vi "Poly_One_Text_Get.vi"(6 "Password?":bool, 7 "Text":string caption="Input Text", 8 "error in":errorcluster, 9 "Button 2 Text":string, 10 "Button 1 Text":string, 11 "Message":string) -> (0 "error out":errorcluster, 2 "Text Out":string caption="Input Text", 3 "Indicator 1":bool)   [LabVIEW 2024, in "Launcher_DTU.lvlib"]
uses:
  Launcher_DTU.lvlib
panel:
  out "Message":string
  in  "Button 2":bool
  in  "Button 1":bool
  # "User Input"
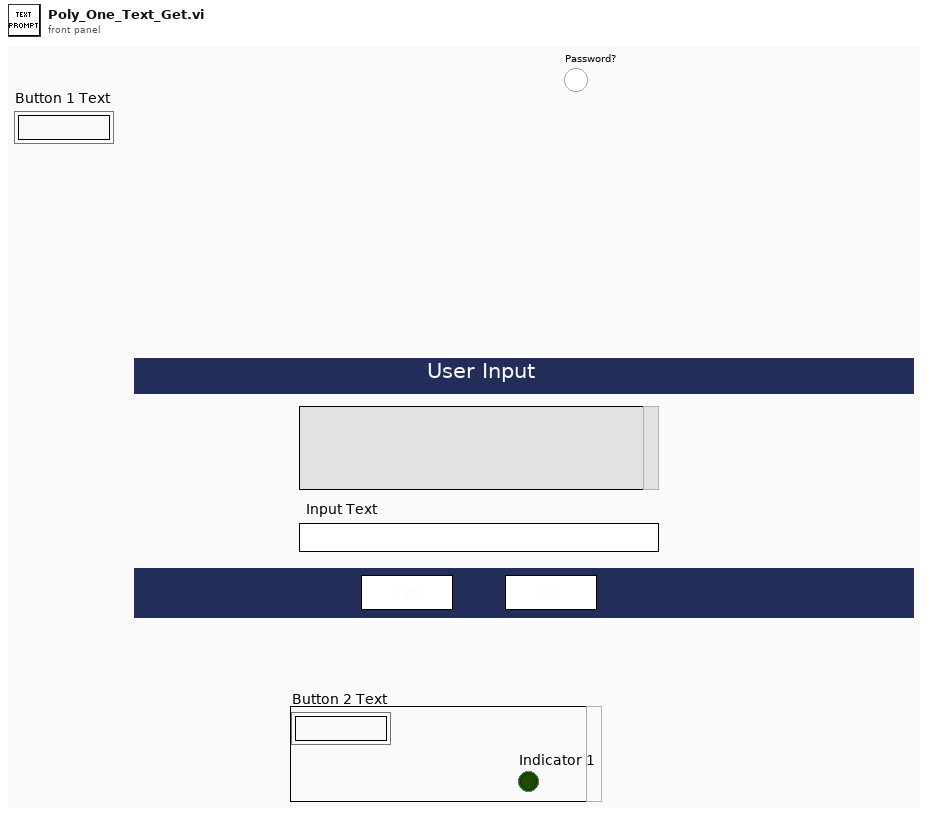
[diagram p1: front panel]
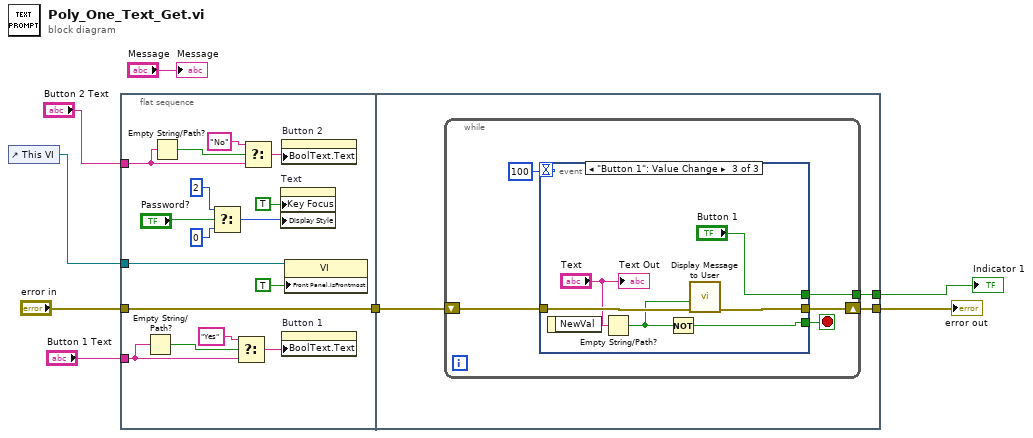
[diagram p0: block diagram]
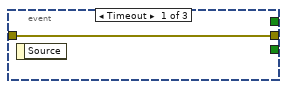
[diagram p2: hidden frame]
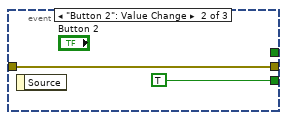
[diagram p3: hidden frame]
diagram:
  n1 = control-ref of="This VI"() -> (w1:refnum<vi>)
  n2 = flat-sequence {
    tunnel: [w24] -> w7
    tunnel: "error in" -> [w24]
    tunnel: "Button 1 Text" -> [w22]
    tunnel: "Button 2 Text" -> [w16]
    tunnel: w1 -> [w14]
    tunnel: [w27] -> w8
    tunnel: w7 -> [w26]
    tunnel: [w25] -> w4
    frame #0 {
      n3 = Empty String/Path?(string/path=w22) -> (empty?=w23:bool)
      n4 = Empty String/Path?(string/path=w16) -> (empty?=w18:bool)
      n5 = Select(t=u32 2 ("Display Style"), s="Password?", f=u32 0 ("Display Style")) -> (s? t:f=w9:u32)
      n6 = Select(t="Yes", s=w23, f=w22) -> (s? t:f=w21:string)
      n7 = Select(t="No", s=w18, f=w16) -> (s? t:f=w17:string)
      n8 = property on="Text" class="Str"("Key Focus"=TRUE, "Display Style"=w9) -> ()  [unwired: 2 in, 2 out]
      n9 = property on="Button 2" class="Bool"("BoolText.Text"=w17) -> ()  [unwired: 2 in, 2 out]
      n10 = property on="Button 1" class="Bool"("BoolText.Text"=w21) -> ()  [unwired: 2 in, 2 out]
      n11 = property class="VI"(reference=w14, "Front Panel.IsFrontmost"=TRUE ("Key Focus")) -> ()  [unwired: 1 in, 2 out]
    }
    frame #1 {
      n12 = while {
        shift-right: [w30] -> w27
        shift-left: w26 -> [w31]
        tunnel: [w29] -> w25
        stop <- w28 stop-if-true
        n13 = event shown="[2] \"Button 1\": Value Change" {
          selector: _ -> [_ _ _]
          dyn-events: _ -> [_ _ _]
          timeout: 100 -> [_ _ _]
          tunnel: [_ TRUE w40] -> w28
          tunnel: w31 -> [w33 w35 w39]
          tunnel: [w33 w35 w38] -> w30
          tunnel: [_ _ "Button 1"] -> w29
          event Timeout {
            n14 = event-data() -> ()  [unwired: 1 in, 1 out]
          }
          event "Button 2": Value Change {
            n15 = event-data() -> ()  [unwired: 1 in, 1 out]
          }
          event "Button 1": Value Change {
            n16 = event-data() -> ()  [unwired: 1 in, 1 out]
            n17 = Empty String/Path?(string/path="Text") -> (empty?=w37:bool)
            n18 = Not(x=w37) -> (.not. x?=w40:bool)
            n19 = call "Display Message to User"("error in (no error)"=w39, "Enable"=w37) -> ("error out"=w38:errorcluster)  [unwired: 8 in, 1 out]
            "Text Out" <- "Text"
          }
        }
      }
    }
  }
  "error out" <- w8
  "Indicator 1" <- w4
  "Message" <- "Message"
